vi "Generate File Name.vi"(11 "File Obs in":refnum<class "File Observer.lvclass">) -> (2 "File Name":string, 3 "File Obs out":refnum<class "File Observer.lvclass">)   [LabVIEW 2014, in "File Observer.lvclass"]
doc: "This is the default behavior of the File Observer Class - generate a file name of the format 'pfYYYYMMDD_HHMMSSext' where pf is the File Prefix and ext is the File Extension, both specified by the caller. This VI may be overridden to provide customized functionality."
uses:
  File Observer.lvclass
  File Observer.lvclass/File Observer.ctl
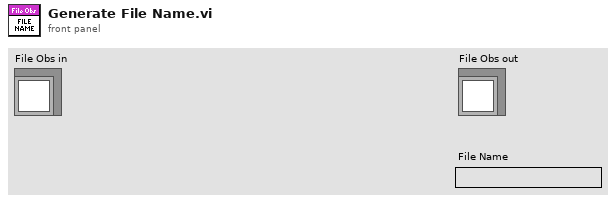
[diagram p1: front panel]
types:
  T1 = typedef "LVDateTimeRec.ctl" = cluster{"fractional second":dbl, "second":i32, "minute":i32, "hour":i32, "day of month":i32, "month":i32, "year":i32, "day of week":i32, "day of year":i32, "DST":i32}
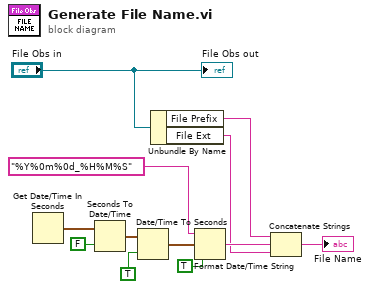
[diagram p0: block diagram]
diagram:
  n1 = Get Date/Time In Seconds() -> (seconds since 1Jan1904=w9:timestamp)
  n2 = Seconds To Date/Time(time stamp (now)=w9, to UTC (F)=FALSE) -> (date time rec=w6:T1)
  n3 = Date/Time To Seconds(1:TRUE ("is UTC (F)"), 2:w6) -> (0:w5:timestamp)
  n4 = Unbundle By Name("File Obs in") -> ("File Prefix"=w1:string, "File Ext"=w4:string)
  n5 = Format Date/Time String(time format string (%c)="%Y%0m%0d_%H%M%S", seconds (now)=w5, UTC format=TRUE) -> (date/time string=w10:string)
  n6 = Concatenate Strings(w1, w10, w4) -> (→"File Name":string)
  "File Obs out" <- "File Obs in"
